vi "GetOperation Name.vi"(8 "error in (no error)":errorcluster caption="entrée d'erreur (pas d'erreur)", 11 "Calculations en entrée":refnum<class "Calculations.lvclass">) -> (0 "error out":errorcluster caption="sortie d'erreur", 2 "Operation Name":string, 3 "Calculations en sortie":refnum<class "Calculations.lvclass">)   [LabVIEW 2019, in "Calculations.lvclass"]
uses:
  Calculations.lvclass
  Calculations.lvclass/Calculations.ctl
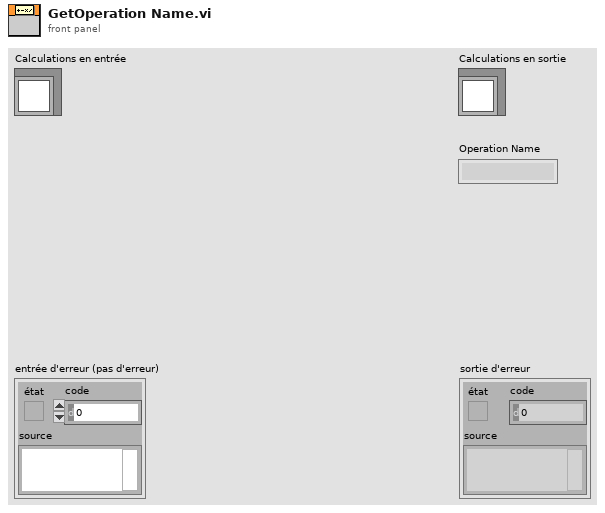
[diagram p1: front panel]
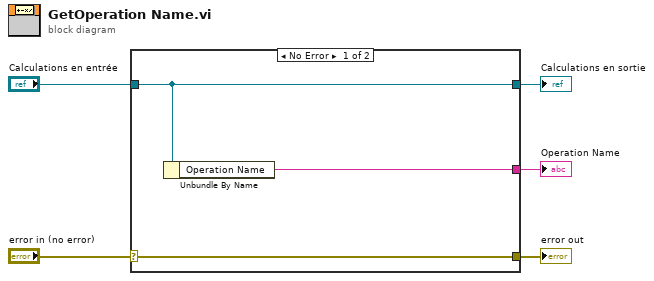
[diagram p0: block diagram]
diagram:
  n1 = case shown="No Error" "error in (no error)" {
    selector: "error in (no error)" -> [w8 w9]
    tunnel: [w8 w9] -> w4
    tunnel: [w7 w10] -> w2
    tunnel: "Calculations en entrée" -> [w7 w10]
    tunnel: [w6 _] -> w1
    frame No Error {
      n2 = Unbundle By Name(w7) -> ("Operation Name"=w6:string)
    }
    frame Error {
    }
  }
  "error out" <- w4
  "Calculations en sortie" <- w2
  "Operation Name" <- w1
